vi "ReadInput.vi"(8 "error in (no error)":errorcluster, 10 "Dynamic data":T1, 11 "Input parameters":T2={"Measurement type"=enum."Debug", "Sensor type"=enum."HPK_8in_256", "Identifier"="test.txt", "Open after execution?"=FALSE, "Plot after execution?"=FALSE, "Display channel"=0, "Voltage Delay (s)"=0.5, "Switch Delay (s)"=0.01, "VISA resource name source"="", "VISA resource name DMM"="", "VISA resource name LCR"="", "Compliance  Level (A)"=10.0, "Voltage Limit (V)"=1000.0, "Data storage location"="", "Scan voltages"="", "Use source as DMM?"=FALSE, "LCR signal frequenzy (Hz)"=10.0, "DMM device"=enum."Keithley2001", "Sampling number"=1, "Use env. sensors on"=enum."Sensirion sht1x/7x", "Switchboard Handle"=0, "Use Switchboard"=FALSE, "LCR signal voltage (V)"=10000.0, "Repeat"=1, "Scan voltages IV"="", "Scan voltages CV"="", "Hex pad numbers?"=FALSE, "Set measurement type"=enum."Debug", "Custom pad scan"="", "IV voltage Delay (s)"=0.5, "CV voltage Delay (s)"=0.5, "Needle measurement?"=FALSE, "Comments"="test.txt", "LCR signal frequenzy (kHz)"=10.0, "Compliance  Level (uA)"=10.0, "Open Correction Array"=array2304x3[6912 elements], "Current set voltage"=0.0, "Last set voltage"=0.0, "Current channel"=0, "Last OpenCorrection index"=-1} {"Last set voltage" format="%#_13g"; "Current set voltage" format="%#_13g"; "CV voltage Delay (s)" format="%#_13g"; "IV voltage Delay (s)" format="%#_13g"; "Voltage Limit (V)" format="%#_13g"; "Voltage Delay (s)" format="%#_13g"; "Switch Delay (s)" format="%#_13g"}) -> (0 "error out":errorcluster, 2 "Dynamic data":T1, 3 "Input parameters":T2={"Measurement type"=enum."Debug", "Sensor type"=enum."HPK_8in_256", "Identifier"="test.txt", "Open after execution?"=FALSE, "Plot after execution?"=FALSE, "Display channel"=0, "Voltage Delay (s)"=0.5, "Switch Delay (s)"=0.01, "VISA resource name source"="", "VISA resource name DMM"="", "VISA resource name LCR"="", "Compliance  Level (A)"=10.0, "Voltage Limit (V)"=1000.0, "Data storage location"="", "Scan voltages"="", "Use source as DMM?"=FALSE, "LCR signal frequenzy (Hz)"=10.0, "DMM device"=enum."Keithley2001", "Sampling number"=1, "Use env. sensors on"=enum."Sensirion sht1x/7x", "Switchboard Handle"=0, "Use Switchboard"=FALSE, "LCR signal voltage (V)"=10000.0, "Repeat"=1, "Scan voltages IV"="", "Scan voltages CV"="", "Hex pad numbers?"=FALSE, "Set measurement type"=enum."Debug", "Custom pad scan"="", "IV voltage Delay (s)"=0.5, "CV voltage Delay (s)"=0.5, "Needle measurement?"=FALSE, "Comments"="test.txt", "LCR signal frequenzy (kHz)"=10.0, "Compliance  Level (uA)"=10.0, "Open Correction Array"=array2304x3[6912 elements], "Current set voltage"=0.0, "Last set voltage"=0.0, "Current channel"=0, "Last OpenCorrection index"=-1} {"Last set voltage" format="%#_13g"; "Current set voltage" format="%#_13g"; "CV voltage Delay (s)" format="%#_13g"; "IV voltage Delay (s)" format="%#_13g"; "Voltage Limit (V)" format="%#_13g"; "Voltage Delay (s)" format="%#_13g"; "Switch Delay (s)" format="%#_13g"})   [LabVIEW 2016]
uses:
  Input_parameters.ctl
  Dynamic_data.ctl
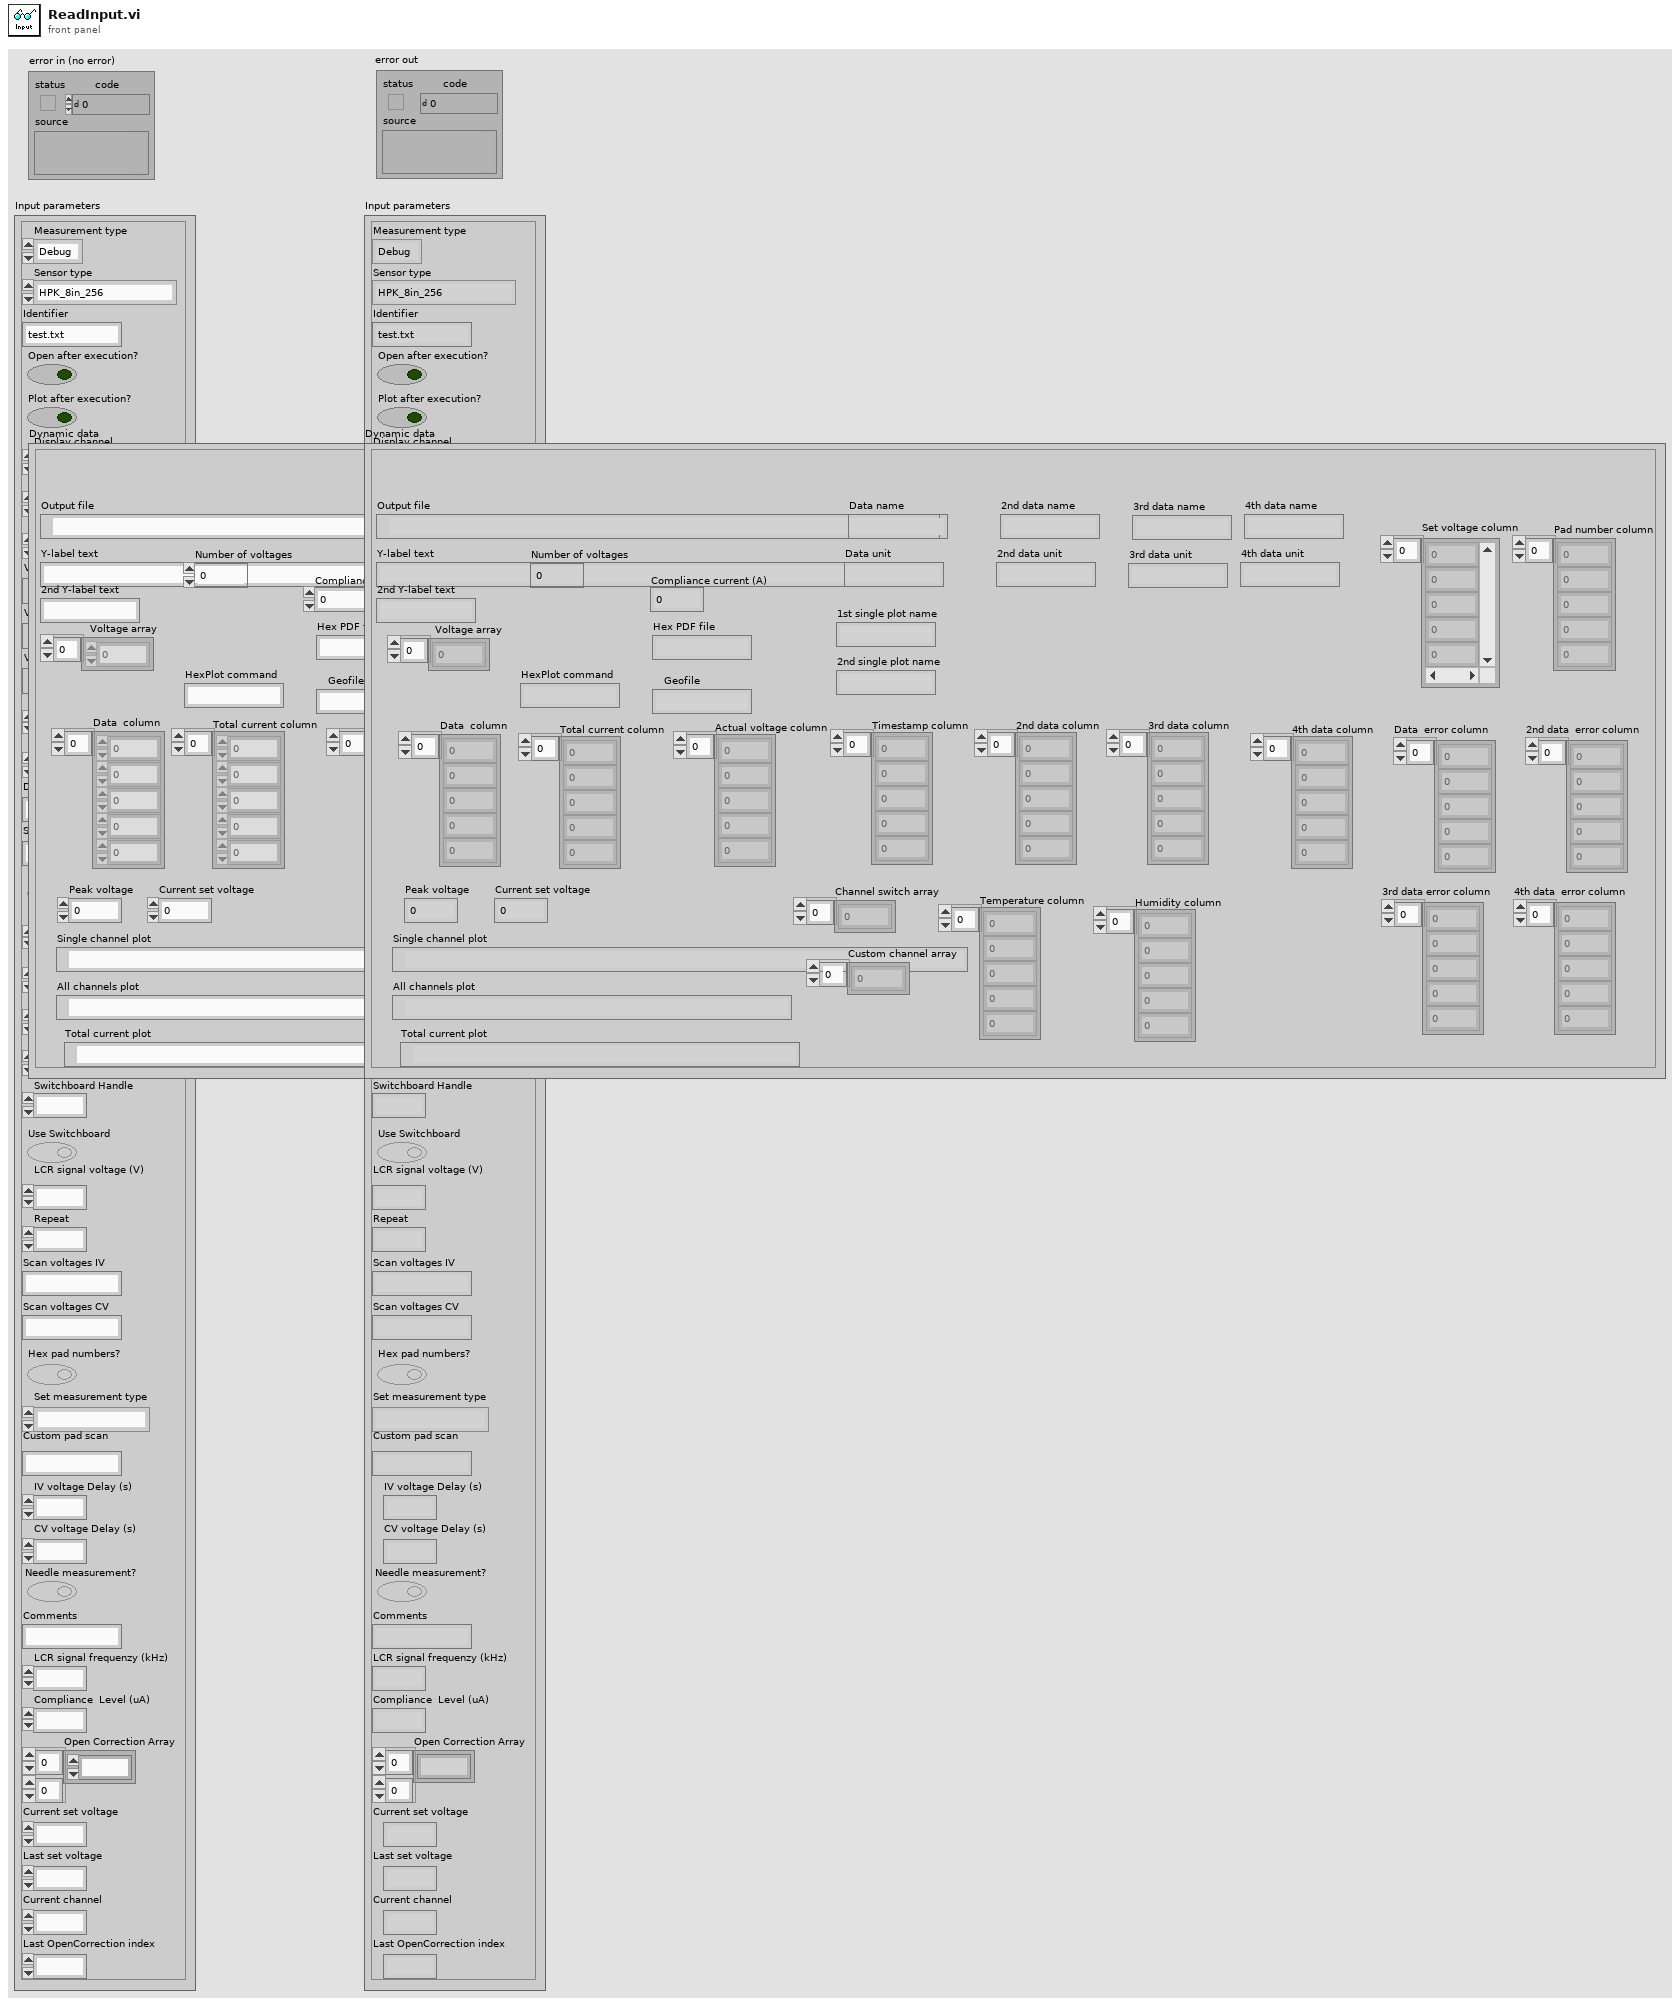
[diagram p1: front panel]
types:
  T1 = typedef "Dynamic_data.ctl" = cluster{"Output file":path, "Y-label text":string, "Current set voltage":dbl, "Set voltage column":dbl[], "Pad number column":dbl[], "Data  column":dbl[], "Number of voltages":i32, "Compliance current (A)":dbl, "Geofile":string, "Peak voltage":dbl, "Hex PDF file":string, "Voltage array":dbl[], "Total current column":dbl[], "Timestamp column":dbl[], "Data name":string, "Data unit":string, "2nd data column":dbl[], "2nd data name":string, "2nd data unit":string, "3rd data column":dbl[], "4th data column":dbl[], "3rd data name":string, "3rd data unit":string, "4th data name":string, "4th data unit":string, "Actual voltage column":dbl[], "2nd Y-label text":string, "Single channel plot":path, "Temperature column":dbl[], "Humidity column":dbl[], "Channel switch array":i32[], "1st single plot name":string, "2nd single plot name":string, "All channels plot":path, "HexPlot command":string, "Custom channel array":i32[], "Data  error column":dbl[], "2nd data  error column":dbl[], "3rd data error column":dbl[], "4th data  error column":dbl[], "Total current plot":path}
  T2 = typedef "Input_parameters.ctl" = cluster{"Measurement type":enum16{"IV", "CV", "Debug", "Test_contact"}, "Sensor type":enum16{"HPK_6in_135", "HPK_8in_256", "INF_8in_256", "Diode", "HPK_6in_256", "Test capacitances", "Full matrix"}, "Identifier":string, "Open after execution?":bool, "Plot after execution?":bool, "Display channel":i32, "Voltage Delay (s)":dbl, "Switch Delay (s)":dbl, "VISA resource name source":refnum<visa-resource-name>, "VISA resource name DMM":refnum<visa-resource-name>, "VISA resource name LCR":refnum<visa-resource-name>, "Compliance  Level (A)":dbl, "Voltage Limit (V)":dbl, "Data storage location":string, "Scan voltages":string, "Use source as DMM?":bool, "LCR signal frequenzy (Hz)":dbl, "DMM device":enum16{"Keithley2001", "Keithley2450", "Keithley2410", "Keithley6487"}, "Sampling number":i32, "Use env. sensors on":enum16{"Sensirion sht1x/7x", "Switch Matrix", "Probecard"}, "Switchboard Handle":u32, "Use Switchboard":bool, "LCR signal voltage (V)":dbl, "Repeat":i32, "Scan voltages IV":string, "Scan voltages CV":string, "Hex pad numbers?":bool, "Set measurement type":enum16{"IV", "CV", "Debug", "Test_contact", "IV+CV"}, "Custom pad scan":string, "IV voltage Delay (s)":dbl, "CV voltage Delay (s)":dbl, "Needle measurement?":bool, "Comments":string, "LCR signal frequenzy (kHz)":dbl, "Compliance  Level (uA)":dbl, "Open Correction Array":dbl[][], "Current set voltage":dbl, "Last set voltage":dbl, "Current channel":i32, "Last OpenCorrection index":i32}
  T3 = enum16{"HPK_6in_135", "HPK_8in_256", "INF_8in_256", "Diode", "HPK_6in_256", "Test capacitances", "Full matrix"}
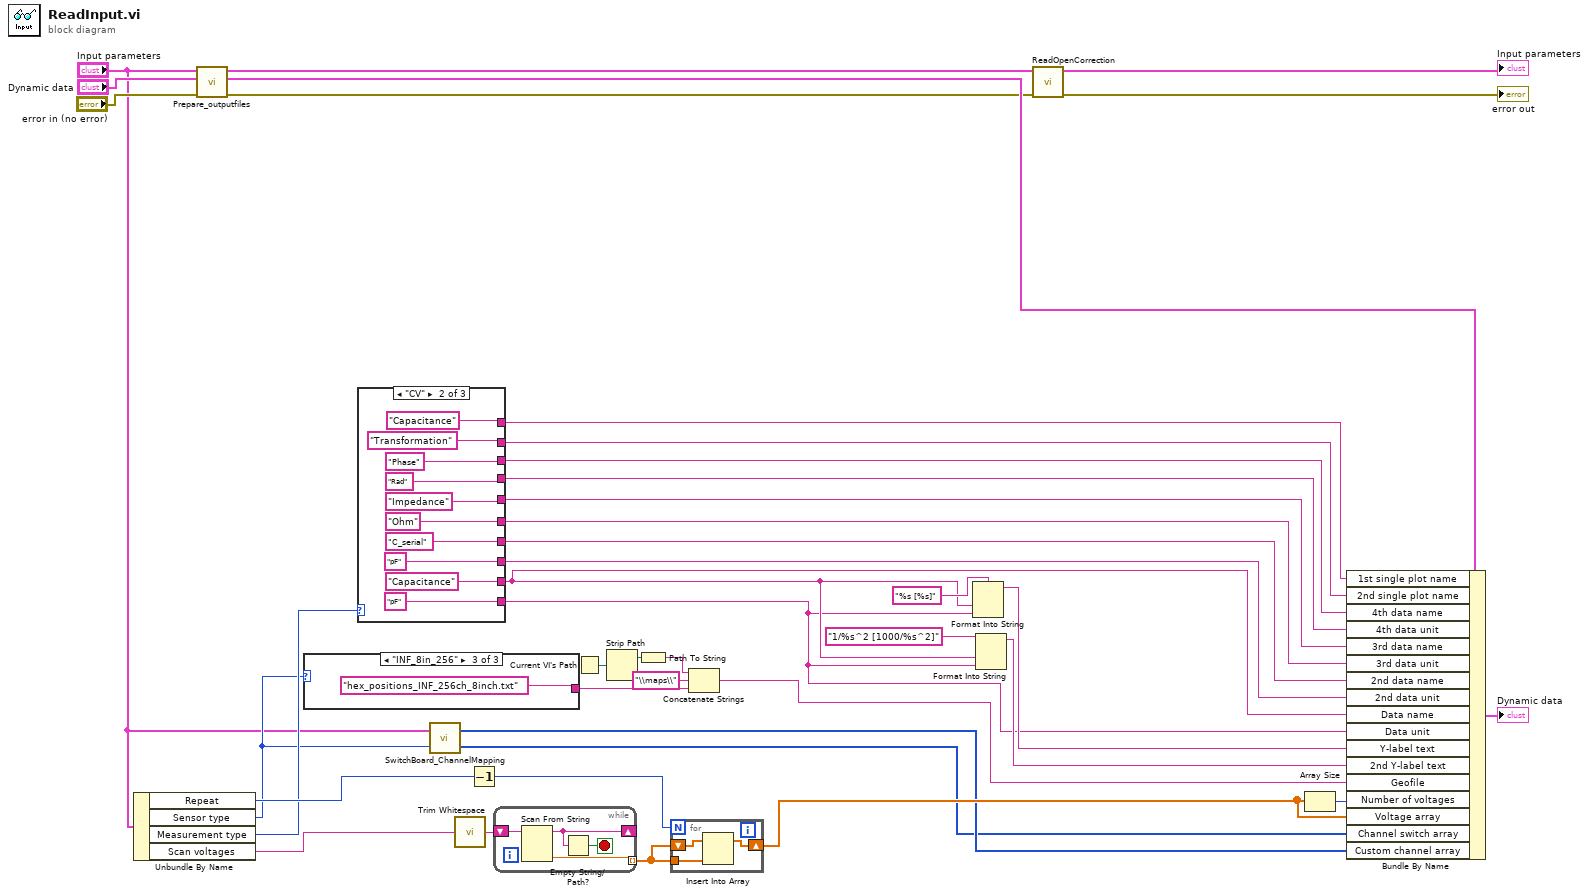
[diagram p0: block diagram]
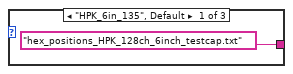
[diagram p2: hidden frame]
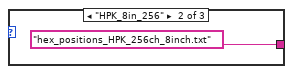
[diagram p3: hidden frame]
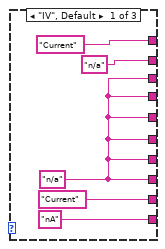
[diagram p4: hidden frame]
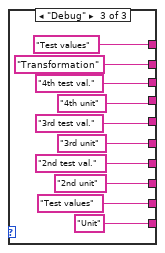
[diagram p5: hidden frame]
diagram:
  n1 = Unbundle By Name("Input parameters") -> ("Repeat"=w22:i32, "Sensor type"=w11:T3, "Measurement type"=w12:enum16{"IV", "CV", "Debug", "Test_contact"}, "Scan voltages"=w16:string)
  n2 = call "Prepare_outputfiles.vi"("error in"="error in (no error)", "Dynamic data in"="Dynamic data", "Input parameters 2"="Input parameters") -> ("error out"=w5:errorcluster, "Dynamic data out"=w13:T1, "Input parameters"=w3:T2)  [unwired: 6 in]
  n3 = case shown="\"INF_8in_256\"" w11 {
    tunnel: ["hex_positions_HPK_128ch_6inch_testcap.txt" "hex_positions_HPK_256ch_8inch.txt" ("name or relative path") "hex_positions_INF_256ch_8inch.txt" ("name or relative path")] -> w39
    frame "HPK_6in_135", Default {
    }
    frame "HPK_8in_256" {
    }
    frame "INF_8in_256" {
    }
  }
  n4 = case shown="\"CV\"" w12 {
    tunnel: ["Current" "Capacitance" "Test values"] -> w25
    tunnel: ["nA" "pF" "Unit"] -> w9
    tunnel: [w46 "C_serial" "2nd test val."] -> w1
    tunnel: [w46 "pF" "2nd unit"] -> w31
    tunnel: [w46 "Ohm" "3rd unit"] -> w30
    tunnel: [w46 "Impedance" "3rd test val."] -> w29
    tunnel: [w46 "Rad" "4th unit"] -> w28
    tunnel: [w46 "Phase" "4th test val."] -> w27
    tunnel: ["Current" "Capacitance" "Test values"] -> w17
    tunnel: ["n/a" "Transformation" "Transformation"] -> w18
    frame "IV", Default {
      w46 = "n/a"
    }
    frame "CV" {
    }
    frame "Debug" {
    }
  }
  n5 = call <instrlib>:"SwitchBoard_ChannelMapping.vi"("Sensor type"=w11, "Input parameters"="Input parameters") -> ("Channel array"=w6:i32[], "Custom pad array"=w7:i32[])
  n6 = call <vilib>:"Trim Whitespace.vi"("string"=w16) -> ("trimmed string"=w36:string)  [unwired: 1 in]
  n7 = Decrement(x=w22) -> (x-1=w20:i32)
  n8 = while {
    shift-right: [w70] -> _
    shift-left: w36 -> [w71]
    tunnel: [w72] -> w21 mode=indexing
    stop <- w69 stop-if-true
    n9 = Scan From String(input string=w71) -> (remaining string=w70:string, output 1=w72:dbl)  [unwired: 4 in, 2 out]
    n10 = Empty String/Path?(string/path=w70) -> (empty?=w69:bool)
  }
  n11 = Current VI's Path() -> (path=w35:path)
  n12 = Strip Path(path=w35) -> (stripped path=w34:path)  [unwired: 1 out]
  n13 = Path To String(path=w34) -> (string=w33:string)
  n14 = for {
    N: w20 -> [_]
    tunnel: w21 -> [w74]
    shift-right: [w73] -> w19
    shift-left: w21 -> [w75]
    n15 = Insert Into Array(array=w75, new element=w74) -> (w73:dbl[])  [unwired: 1 in]
  }
  n16 = Concatenate Strings(w33, "\\maps\\" ("string"), w39) -> (w8:string)
  n17 = Format Into String(format string="%s [%s]", w25, w9) -> (resulting string=w23:string)  [unwired: 2 in, 1 out]
  n18 = Format Into String(format string="1/%s^2 [1000/%s^2]", w25, w9) -> (resulting string=w24:string)  [unwired: 2 in, 1 out]
  n19 = call "ReadOpenCorrection.vi"("error in"=w5, "Input parameters in"=w3) -> ("error out"=→"error out":errorcluster, "Input parameters out"=→"Input parameters":T2)  [unwired: 8 in]
  n20 = Array Size(array=w19) -> (size(s)=w37:i32)
  n21 = Bundle By Name(cluster=w13, "1st single plot name"=w17, "2nd single plot name"=w18, "4th data name"=w27, "4th data unit"=w28, "3rd data name"=w29, "3rd data unit"=w30, "2nd data name"=w1, "2nd data unit"=w31, "Data name"=w25, "Data unit"=w9, "Y-label text"=w23, "2nd Y-label text"=w24, "Geofile"=w8, "Number of voltages"=w37, "Voltage array"=w19, "Channel switch array"=w6, "Custom channel array"=w7) -> (→"Dynamic data":T1)
